vi "Get Data folder path.vi"(8 "error in":errorcluster, 11 "Data Path Name":string="data") -> (0 "error out":errorcluster, 2 "App.Kind":T1(ring), 3 "Data Path":path)   [LabVIEW 2009]
doc: "Ce VI permet de renvoyer le chemin du dossier data. On a 2 cas\n1 Cas-- Systeme de developpement labview.\nSi le dossier data n'existe pas il le crée et renvoye son chemin.\nCependant il si le dossier data existait il renvoye uniquement son chemin.\n\n2 Cas-- Run Time System (Installeur, Excecutable)\nSi le dossier data existe il renvoye son chemin.\nSi le dossier data n'existe pas il renvoye un message d'erreur et quitte le systeme."
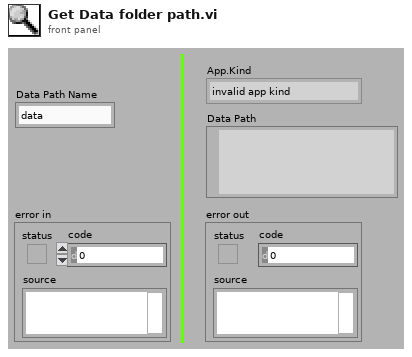
[diagram p1: front panel]
types:
  T1 = enum32{"invalid app kind", "Development System", "Run Time System", "Student Edition", "Embedded LabVIEW", "Evaluation", "Custom"}
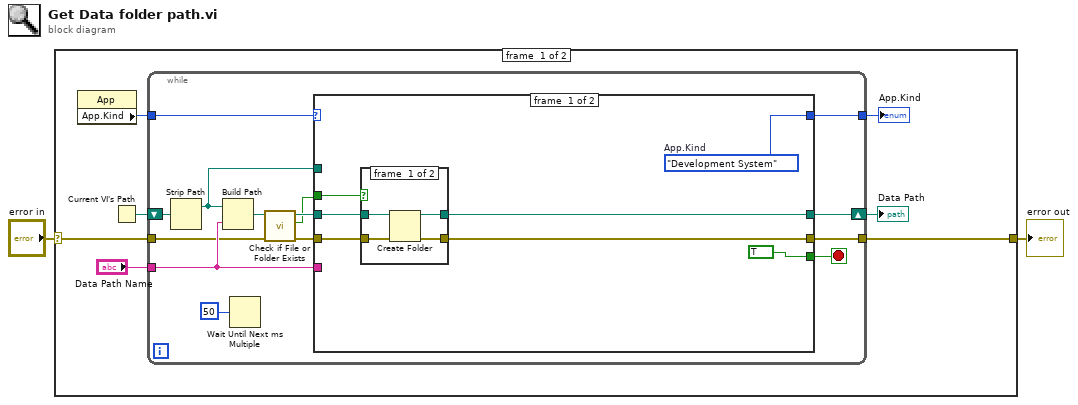
[diagram p0: block diagram]
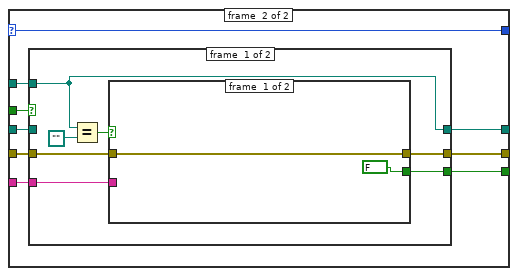
[diagram p3: hidden frame]
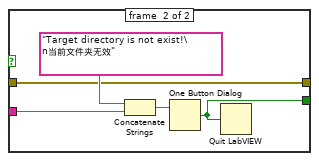
[diagram p4: hidden frame]
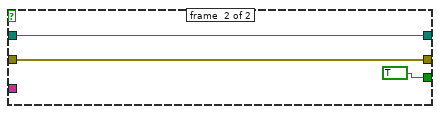
[diagram p5: hidden frame]
diagram:
  n1 = case shown="No Error" "error in" {
    selector: "error in" -> [w4 w63]
    tunnel: [w5 w63] -> w1
    frame #0 {
      n2 = property class="App"() -> ("App.Kind"=w9:T1)  [unwired: 2 in, 2 out]
      n3 = Current VI's Path() -> (path=w8:path)
      n4 = while {
        shift-right: [w15] -> w6
        shift-left: w8 -> [w23]
        tunnel: "Data Path Name" -> [w20]
        tunnel: w9 -> [w19]
        tunnel: [w12] -> w5
        tunnel: w4 -> [w11]
        tunnel: [w10] -> w3
        stop <- w17 stop-if-true
        n5 = Strip Path(path=w23) -> (stripped path=w14:path)  [unwired: 1 out]
        n6 = Build Path(base path=w14, name or relative path=w20) -> (appended path=w21:path)
        n7 = Wait Until Next ms Multiple(millisecond multiple=u32 50 ("n millisecondes")) -> ()  [unwired: 1 out]
        n8 = call <vilib>:"Check if File or Folder Exists.vi"("error in (no error)"=w11, "path"=w21) -> ("error out"=w13:errorcluster, "file or folder exists?"=w16:bool, "dup path"=w18:path)  [unwired: 7 out]
        n9 = case shown="\"Run Time System\"" w19 {
          selector: w19 -> [_ w37]
          tunnel: w16 -> [w30 w45]
          tunnel: w20 -> [_ w44]
          tunnel: w18 -> [w29 w42]
          tunnel: [w28 w43] -> w15
          tunnel: [TRUE w41] -> w17
          tunnel: w14 -> [_ w40]
          tunnel: w13 -> [w26 w38]
          tunnel: [w25 w39] -> w12
          tunnel: [w24 w37] -> w10
          frame #0 {
            w24 = T1."Development System"  # App.Kind
            n10 = case shown="False" w30 {
              tunnel: [w33 w36] -> w28
              tunnel: w29 -> [w34 w36]
              tunnel: w26 -> [w32 w35]
              tunnel: [w31 w35] -> w25
              frame #0 {
                n11 = Create Folder(path (use dialog)=w34, error in=w32) -> (created path=w33:path, error out=w31:errorcluster)  [unwired: 2 out]
              }
              frame #1 {
              }
            }
          }
          frame #1 {
            n12 = case shown="False" w45 {
              tunnel: w44 -> [w48 _]
              tunnel: [w51 w62] -> w43
              tunnel: w42 -> [_ w62]
              tunnel: [w49 TRUE] -> w41
              tunnel: w40 -> [w51 _]
              tunnel: [w47 w60] -> w39
              tunnel: w38 -> [w46 w60]
              frame #0 {
                n13 = Equal?(x=w51, y=path "") -> (x = y?=w50:bool)
                n14 = case shown="True" w50 {
                  tunnel: [FALSE w57] -> w49
                  tunnel: w48 -> [_ w58]
                  tunnel: [w53 w55] -> w47
                  tunnel: w46 -> [w53 w55]
                  frame #0 {
                  }
                  frame #1 {
                    n15 = Concatenate Strings("Target directory is not exist!\n当前文件夹无效" ("message"), w58) -> (w56:string)
                    n16 = One Button Dialog(message=w56) -> (true=w57:bool)  [unwired: 1 out]
                    n17 = Quit LabVIEW(quit? (T)=w57) -> ()
                  }
                }
              }
              frame #1 {
              }
            }
          }
        }
      }
      "Data Path" <- w6
      "App.Kind" <- w3
    }
    frame #1 {
    }
  }
  "error out" <- w1
